vi "ueye array to image.vi"(8 "Error In":errorcluster, 9 "Image In":T1, 10 "InArray":u8[](array[numeric]), 11 "Camera Reference":refnum<k24>) -> (0 "Error Out":errorcluster, 1 "Image Out":T1, 3 "Camera reference out":refnum<k24>)   [LabVIEW 2022 SP3, in "Vision.lvlib"]
doc: "ArrayToVision converts 24/32-bit one-dimensional arrays to a two-dimensional U32 array."
uses:
  Vision.lvlib
  C:/Users/Caleb/Desktop/nebraska-silicon-lab/pixel-gantry-control/Gantry/Shared Components/bin/uEyeDotNet.dll
  bin/uEyeDotNet.dll
  <vilib>/vision/Image Controls.llb/IMAQ Image.ctl
panel:
  # "Output"
  # "Input"
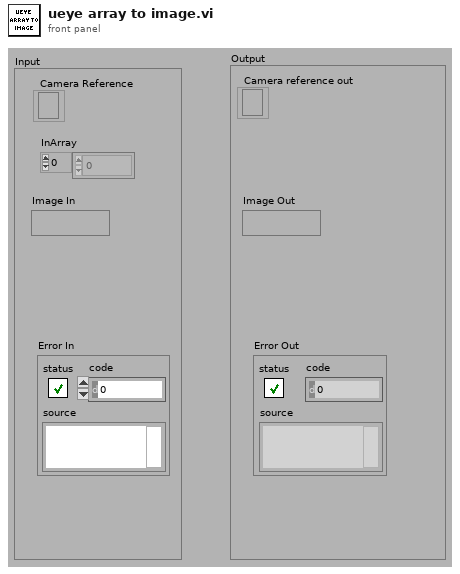
[diagram p1: front panel]
types:
  T1 = typedef "IMAQ Image.ctl" = refnum<image>
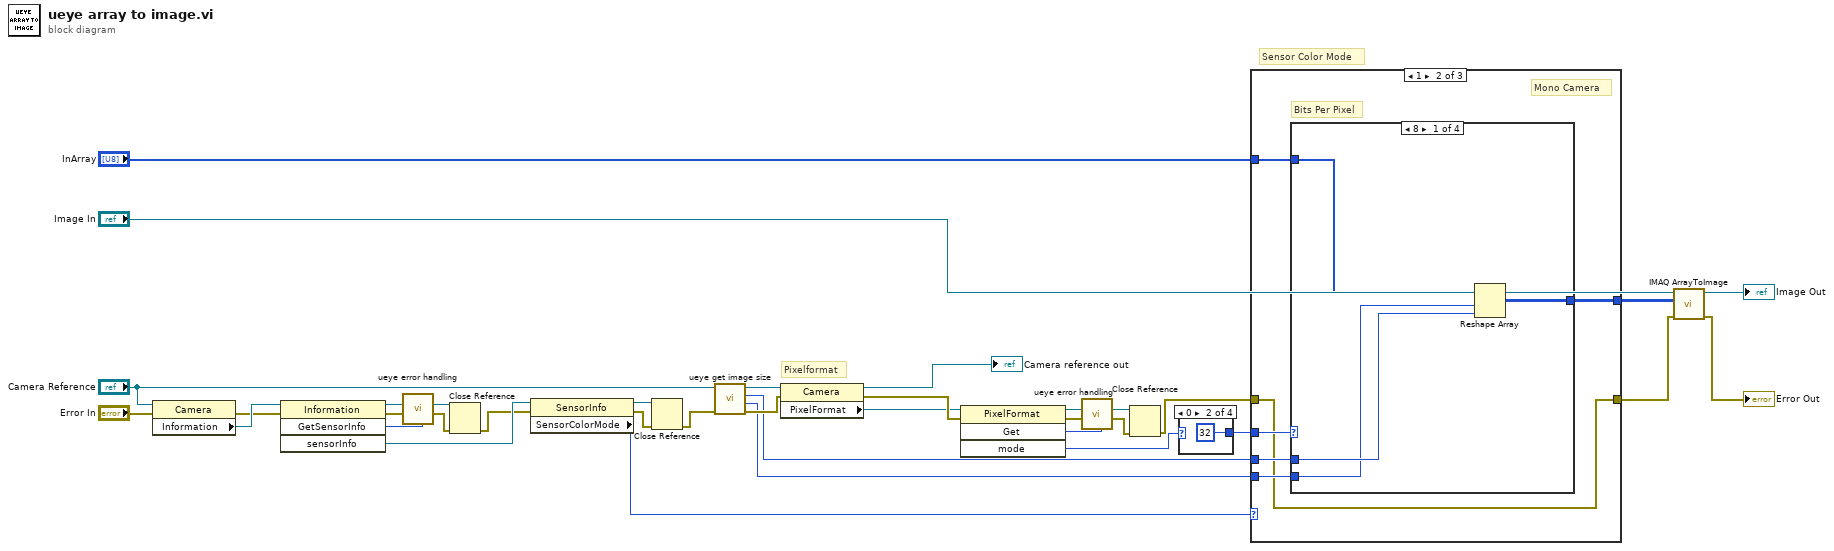
[diagram p0: block diagram]
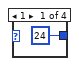
[diagram p2: hidden frame]
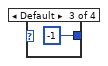
[diagram p3: hidden frame]
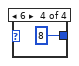
[diagram p4: hidden frame]
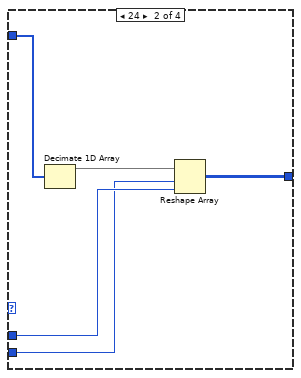
[diagram p6: hidden frame]
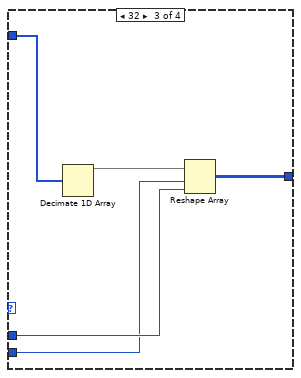
[diagram p7: hidden frame]
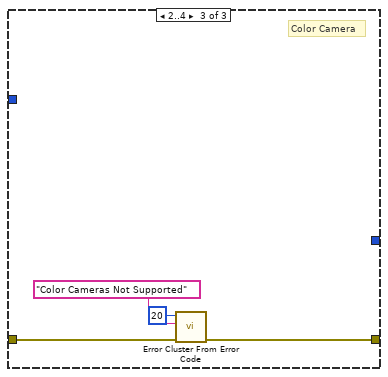
[diagram p9: hidden frame]
diagram:
  # "Sensor Color Mode"
  # "Pixelformat"
  n1 = property on="Eigenschaftsknoten" class="Camera"(reference="Camera Reference", error in="Error In") -> (error out=w31:errorcluster, "Information"=w34:refnum<k24>)  [unwired: 1 out]
  n2 = invoke class="Information" method="GetSensorInfo"(reference=w34, error in=w31) -> (reference out=w9:refnum<k24>, error out=w14:errorcluster, "GetSensorInfo"=w13:i32, "sensorInfo"=w33:refnum<k24>)  [unwired: 2 in]
  n3 = call "ueye error handling.vi"("Error Code"=w13, "reference in"=w9, "Error In"=w14) -> ("Error Out"=w8:errorcluster)  [unwired: 8 in]
  n4 = Close Reference(reference=w9, error in (no error)=w8) -> (error out=w7:errorcluster)
  n5 = property class="SensorInfo"(reference=w33, error in=w7) -> (reference out=w6:refnum<k24>, error out=w5:errorcluster, "SensorColorMode"=w32:i32)
  n6 = Close Reference(reference=w6, error in (no error)=w5) -> (error out=w4:errorcluster)
  n7 = call "ueye get image size.vi"("Error In"=w4, "Camera reference in"="Camera Reference") -> ("Error Out"=w22:errorcluster, "Height"=w20:i32, "Width"=w21:i32, "Camera reference out"=w23:refnum<k24>)  [unwired: 6 in]
  n8 = property class="Camera"(reference=w23, error in=w22) -> (reference out=→"Camera reference out":refnum<k24>, error out=w28:errorcluster, "PixelFormat"=w27:refnum<k24>)
  n9 = invoke class="PixelFormat" method="Get"(reference=w27, error in=w28) -> (reference out=w3:refnum<k24>, error out=w12:errorcluster, "Get"=w11:i32, "mode"=w26:i32)  [unwired: 2 in]
  n10 = call "ueye error handling.vi"("Error Code"=w11, "reference in"=w3, "Error In"=w12) -> ("Error Out"=w2:errorcluster)  [unwired: 8 in]
  n11 = Close Reference(reference=w3, error in (no error)=w2) -> (error out=w1:errorcluster)
  n12 = case shown="0" w26 {
    tunnel: [24 32 -1 8] -> w25
    frame 1 {
    }
    frame 0 {
    }
    frame Default {
    }
    frame 6 {
    }
  }
  n13 = case shown="1" w32 {
    tunnel: "InArray" -> [_ w45 _]
    tunnel: w21 -> [_ w43 _]
    tunnel: w20 -> [_ w42 _]
    tunnel: w25 -> [_ w44 _]
    tunnel: [w39 w40 w63] -> w18
    tunnel: [_ w41 _] -> w19
    tunnel: w1 -> [w39 w40 w60]
    frame 0, Default {
    }
    frame 1 {
      # "Bits Per Pixel"
      # "Mono Camera"
      n14 = case shown="8" w44 {
        tunnel: w45 -> [w46 w54 w58 _]
        tunnel: w42 -> [w47 w51 w56 _]
        tunnel: w43 -> [w48 w52 w57 _]
        tunnel: [w49 w53 w59 _] -> w41
        frame 8 {
          n15 = Reshape Array(w46, w47, w48) -> (w49:u8[][])
        }
        frame 24 {
          n16 = Decimate 1D Array(w54) -> (w50:u8[])  [unwired: 2 out]
          n17 = Reshape Array(w50, w51, w52) -> (w53:u8[][])
        }
        frame 32 {
          n18 = Decimate 1D Array(w58) -> (w55:u8[])  [unwired: 3 out]
          n19 = Reshape Array(w55, w56, w57) -> (w59:u8[][])
        }
        frame Default {
        }
      }
    }
    frame 2..4 {
      # "Color Camera"
      n20 = call <vilib>:"Error Cluster From Error Code.vi"("error in (no error)"=w60, "error message (\"\")"="Color Cameras Not Supported" ("error message (\"\")"), "error code (0)"=20) -> ("error out"=w63:errorcluster)  [unwired: 6 in]
    }
  }
  n21 = call "IMAQ ArrayToImage"("error in (no error)"=w18, "Image Pixels (U8)"=w19, "Image"="Image In") -> ("error out"=→"Error Out":errorcluster, "Image Out"=→"Image Out":T1)  [unwired: 7 in]
